vi "Temperatury.vi"() -> ()   [LabVIEW 2020]
panel:
  out "Waveform Graph":cluster{dbl, dbl, dbl[]}(graph)
  out "Sweep mode Chart":cluster{"Thermometer":dbl, "Numeric":dbl}(graph)
  out "Scope mode Chart":cluster{"Numeric":dbl, "Thermometer":dbl}(graph)
  out "Strip Mode Chart":cluster{"Thermometer":dbl, dbl}(graph)
  in  "Aby wyœwietliæ zebrane dane zatrzymaj program":bool
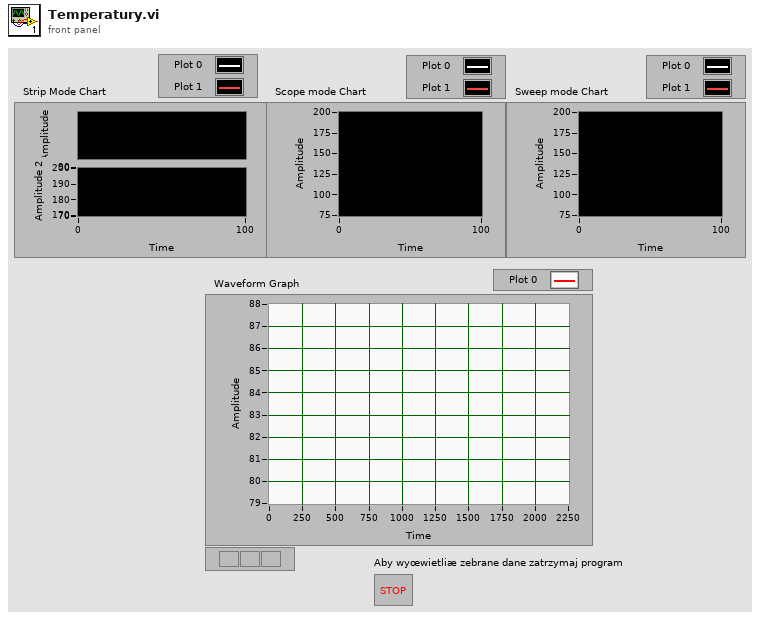
[diagram p1: front panel]
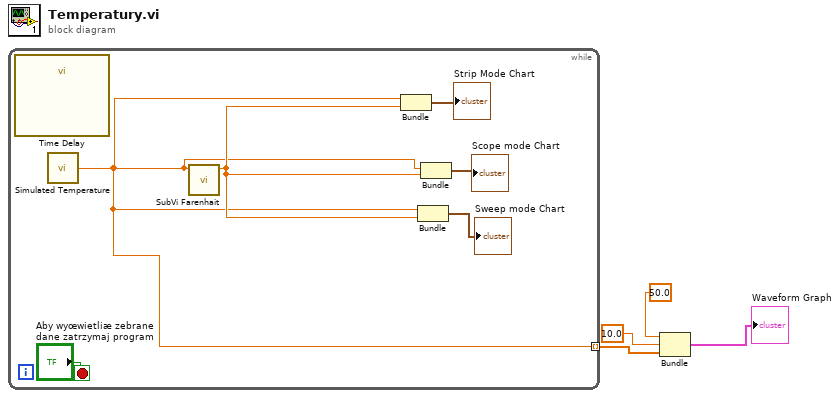
[diagram p0: block diagram]
diagram:
  n1 = while {
    tunnel: [w5] -> w4 mode=indexing
    stop <- "Aby wyœwietliæ zebrane dane zatrzymaj program" stop-if-true
    n2 = call "Time Delay"() -> ()  [unwired: 11 in, 1 out]
    n3 = call "Simulated Temperature.vi"() -> ("Thermometer"=w5:dbl)  [unwired: 1 in]
    n4 = call "SubVi Farenhait.vi"("Thermometer"=w5) -> ("Numeric"=w6:dbl)  [unwired: 10 in]
    n5 = Bundle("Thermometer"=w5, "Numeric"=w6) -> (→"Strip Mode Chart":cluster{"Thermometer":dbl, "Numeric":dbl})  [unwired: 1 in]
    n6 = Bundle("Thermometer"=w5, "Numeric"=w6) -> (→"Sweep mode Chart":cluster{"Thermometer":dbl, "Numeric":dbl})  [unwired: 1 in]
    n7 = Bundle("Thermometer"=w5, "Numeric"=w6) -> (→"Scope mode Chart":cluster{"Thermometer":dbl, "Numeric":dbl})  [unwired: 1 in]
  }
  n8 = Bundle(50.0, 10.0, w4) -> (→"Waveform Graph":cluster{dbl, dbl, dbl[]})  [unwired: 1 in]
